vi "Example Callback - Humidity Callback.vi"(4 "Humidity":refnum<user-event>, 5 "Event Data":cluster{"sender":refnum<k24>, "humidity":i32}, 6 "Control Ref":refnum<k24>, 7 "Event Common Data":T1) -> ()   [LabVIEW 2013]
uses:
  C:/tf/play/labview/Tinkerforge.dll
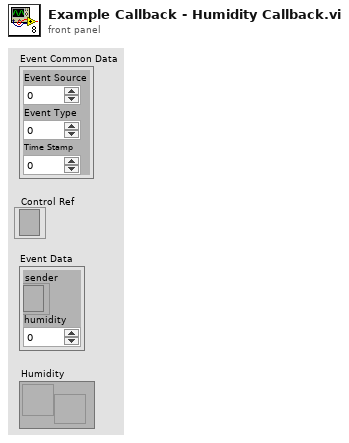
[diagram p1: front panel]
types:
  T1 = cluster{"Event Source":i32, "Event Type":u32, "Time Stamp":u32}
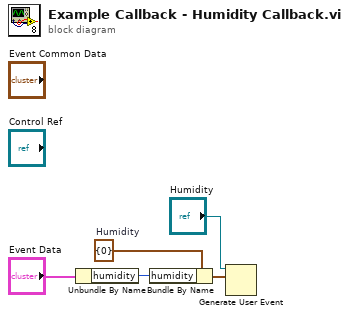
[diagram p0: block diagram]
diagram:
  w3 = cluster{"humidity":i32} {"humidity"=0}  # Humidity
  n1 = Unbundle By Name("Event Data") -> ("humidity"=w4:i32)
  n2 = Bundle By Name(cluster=w3, "humidity"=w4) -> (w2:cluster{"humidity":i32})
  n3 = Generate User Event(user event="Humidity", event data cluster=w2) -> ()  [unwired: 2 in, 2 out]
